vi "Test Scale Line Segment.vi"() -> ()   [LabVIEW 2011]
uses:
  Vec3d Class/Vec3d Class.lvclass
panel:
  in  "Scale Factor":dbl=1.0
  out "Point B out":cluster{"X":dbl, "Y":dbl, "Z":dbl}
  out "Point A out":cluster{"X":dbl, "Y":dbl, "Z":dbl}
  in  "Point B in":cluster{"X":dbl, "Y":dbl, "Z":dbl}
  in  "Point A in":cluster{"X":dbl, "Y":dbl, "Z":dbl}
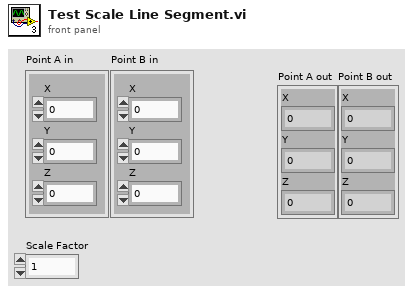
[diagram p1: front panel]
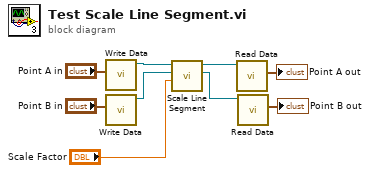
[diagram p0: block diagram]
diagram:
  n1 = call "Write Data.vi"("Data"="Point A in") -> ("Vec3d Class out"=w9:refnum<class "Vec3d Class.lvclass">)  [unwired: 9 in, 1 out]
  n2 = call "Write Data.vi"("Data"="Point B in") -> ("Vec3d Class out"=w8:refnum<class "Vec3d Class.lvclass">)  [unwired: 9 in, 1 out]
  n3 = call "Scale Line Segment.vi"("Scale Factor"="Scale Factor", "Point B in"=w8, "Point A in"=w9) -> ("Point B out"=w4:refnum<class "Vec3d Class.lvclass">, "Point A out"=w5:refnum<class "Vec3d Class.lvclass">)  [unwired: 6 in, 1 out]
  n4 = call-dynamic "Read Data.vi"("Vec3d Class in"=w5) -> ("Data"=→"Point A out":cluster{"X":dbl, "Y":dbl, "Z":dbl})  [unwired: 8 in, 2 out]
  n5 = call-dynamic "Read Data.vi"("Vec3d Class in"=w4) -> ("Data"=→"Point B out":cluster{"X":dbl, "Y":dbl, "Z":dbl})  [unwired: 8 in, 2 out]
